vi "Teste-Circulos.vi"() -> ()   [LabVIEW 2014]
doc: "Newport Motion Controler\nThis VI test a Group\n\nAndré Romero - 2022\nandretec@ifsc.usp.br"
uses:
  <vilib>/Platform/TimedLoop/XDataNode/timing_clust.ctl
  <vilib>/Platform/TimedLoop/XDataNode/nitl_modes.ctl
  <vilib>/Platform/TimedLoop/XDataNode/wakeup.ctl
  <vilib>/Platform/TimedLoop/XDataNode/XDataNode.xnode
  <userlib>/Newport ESP301/Newport ESP301.lvlib
  <vilib>/Platform/TimedLoop/XDataNode/XDNodeRunTimeDep.lvlib
panel:
  out "Position (units) 4":dbl format="%.6g"
  out "Position (units) 3":dbl format="%.6g"
  out "Position (units) 2":dbl format="%.6g"
  out "Position (units)":dbl format="%.6g"
  in  "arc sweep angle":dbl=360.0 format="%#_13g"
  in  "Second coordonate of arc center":dbl format="%#_13g"
  in  "first coordonate of arc":dbl=0.1 format="%#_13g"
  in  "Stop Button":bool
  out "error out":errorcluster
  out "Y":dbl format="%.2g"
  out "X":dbl=-0.2115 format="%.2f"
  out "XY Graph":cluster{dbl[], dbl[]}(graph)={[-0.0005, -0.027, -0.0515, -0.076, -0.1, -0.1235, -0.146, -0.1675, -0.1885, -0.207, -0.2255, -0.242, -0.257, -0.2705, -0.2815, -0.2915, -0.2995, -0.3055, -0.3095, -0.3115, -0.312, -0.311, -0.3055, -0.2995, -0.292, -0.282, -0.2705, -0.257, -0.242, -0.2255, -0.2075, -0.1885, -0.168, -0.146, -0.1235, -0.1005, -0.076, -0.052, -0.0275, -0.0025, 0.023, 0.0475, 0.0725, 0.0965, 0.1195, 0.142, 0.164, 0.185, 0.204, 0.2225, 0.239, 0.2545, 0.268, 0.2795, 0.2895, 0.2975, 0.3045, 0.3085, 0.311, 0.3115, 0.311, 0.3065, 0.3, 0.2925, 0.283, 0.2715, 0.2585, 0.244, 0.2275, 0.2095, 0.191, 0.1705, 0.149, 0.126, 0.1035, 0.079, 0.0545, 0.03, 0.0055, -0.0015, -0.0005, 0.0, 0.0, 0.0, 0.0, 0.0, 0.0, 0.0, 0.0, 0.0, 0.0, 0.0, 0.0, 0.0, 0.0, 0.0, 0.0, 0.0, 0.0, 0.0, 0.0, 0.0, 0.0, 0.0, 0.0, 0.0, 0.0, 0.0, 0.0, 0.0, 0.0, 0.0, 0.0, 0.0, 0.0, 0.0, 0.0, 0.0, 0.0, 0.0, 0.0, 0.0, 0.0, 0.0, 0.0, 0.0, 0.0, 0.0, 0.0, 0.0, 0.0, 0.0, 0.0, 0.0, 0.0, 0.0, 0.0, 0.0, 0.0, 0.0, 0.0, 0.0, 0.0, 0.0, 0.0, 0.0, 0.0, 0.0, 0.0, 0.0, 0.0, 0.0, 0.0, 0.0, 0.0, 0.0, 0.0, 0.0, 0.0, 0.0, 0.0, 0.0, 0.0, 0.0, 0.0, 0.0, 0.0, 0.0, 0.0, 0.0, 0.0, 0.0, 0.0, 0.0, 0.0, 0.0, 0.0, 0.0, 0.0, 0.0, 0.0, 0.0, 0.0, 0.0, 0.0, 0.0, 0.0, 0.0, 0.0, 0.0, 0.0, 0.0, 0.0, 0.0, 0.0, 0.0, 0.0, 0.0, 0.0, 0.0, 0.0, 0.0, 0.0, 0.0, 0.0, 0.0, 0.0, 0.0, 0.0, 0.0, 0.0, 0.0, 0.0, 0.0, 0.0, 0.0, 0.0, 0.0, 0.0, 0.0, 0.0, 0.0, 0.0, 0.0, 0.0, 0.0, 0.0, 0.0, 0.0, 0.0, 0.0, 0.0, 0.0, 0.0, 0.0, 0.0, 0.0, 0.0, 0.0, 0.0, 0.0, 0.0, 0.0, 0.0, 0.0, 0.0, 0.0, 0.0, 0.0, 0.0, 0.0, 0.0, 0.0, 0.0, 0.0, 0.0, 0.0, 0.0, 0.0, 0.0, 0.0, 0.0, 0.0, 0.0, 0.0, 0.0, 0.0, 0.0, 0.0, 0.0, 0.0, 0.0, 0.0, 0.0, 0.0, 0.0, 0.0, 0.0, 0.0, 0.0, 0.0, 0.0, 0.0, 0.0, 0.0, 0.0, 0.0, 0.0, 0.0, 0.0, 0.0, 0.0, 0.0, 0.0, 0.0, 0.0, 0.0, 0.0, 0.0, 0.0, 0.0, 0.0, 0.0, 0.0, 0.0, 0.0, 0.0, 0.0, 0.0, 0.0, 0.0, 0.0, 0.0, 0.0, 0.0, 0.0, 0.0, 0.0, 0.0, 0.0, 0.0, 0.0, 0.0, 0.0, 0.0, 0.0, 0.0, 0.0, 0.0, 0.0, 0.0, 0.0, 0.0, 0.0, 0.0, 0.0, 0.0, 0.0, 0.0, 0.0, 0.0, 0.0, 0.0, 0.0, 0.0, 0.0, 0.0, 0.0, 0.0, 0.0, 0.0, 0.0, 0.0, 0.0, 0.0, 0.0, 0.0, 0.0, 0.0, 0.0, 0.0, 0.0, 0.0, 0.0, 0.0, 0.0, 0.0], [-0.2115, -0.211, -0.2075, -0.202, -0.195, -0.1855, -0.175, -0.1625, -0.148, -0.132, -0.115, -0.096, -0.0765, -0.055, -0.033, -0.01, 0.0135, 0.038, 0.0625, 0.0875, 0.1125, 0.1375, 0.1625, 0.1865, 0.21, 0.233, 0.2555, 0.2765, 0.2965, 0.3155, 0.3325, 0.349, 0.363, 0.3755, 0.386, 0.3955, 0.4025, 0.4075, 0.4105, 0.412, 0.412, 0.41, 0.4035, 0.3965, 0.3875, 0.3775, 0.365, 0.351, 0.3355, 0.318, 0.2995, 0.2795, 0.2585, 0.2365, 0.214, 0.19, 0.166, 0.1415, 0.1165, 0.0915, 0.0665, 0.042, 0.0175, -0.007, -0.0295, -0.0515, -0.073, -0.093, -0.112, -0.13, -0.146, -0.1605, -0.173, -0.184, -0.1935, -0.201, -0.2065, -0.2095, -0.2115, -0.2115, -0.2115, -0.2115, -0.2115, -0.2115, -0.2115, -0.2115, -0.212, -0.2115, -0.2115, -0.2115, -0.2115, -0.2115, -0.2115, -0.2115, -0.2115, -0.2115, -0.2115, -0.2115, -0.2115, -0.2115, -0.2115, -0.2115, -0.2115, -0.2115, -0.2115, -0.2115, -0.2115, -0.2115, -0.2115, -0.2115, -0.2115, -0.2115, -0.2115, -0.2115, -0.2115, -0.2115, -0.2115, -0.2115, -0.2115, -0.2115, -0.2115, -0.2115, -0.2115, -0.2115, -0.2115, -0.2115, -0.2115, -0.2115, -0.2115, -0.2115, -0.2115, -0.2115, -0.2115, -0.2115, -0.2115, -0.2115, -0.2115, -0.2115, -0.2115, -0.2115, -0.2115, -0.2115, -0.2115, -0.2115, -0.2115, -0.2115, -0.2115, -0.2115, -0.2115, -0.2115, -0.2115, -0.2115, -0.2115, -0.2115, -0.2115, -0.2115, -0.2115, -0.2115, -0.2115, -0.2115, -0.2115, -0.2115, -0.2115, -0.2115, -0.2115, -0.2115, -0.2115, -0.2115, -0.2115, -0.2115, -0.2115, -0.2115, -0.2115, -0.2115, -0.2115, -0.2115, -0.2115, -0.2115, -0.2115, -0.2115, -0.2115, -0.2115, -0.2115, -0.2115, -0.2115, -0.2115, -0.2115, -0.2115, -0.2115, -0.2115, -0.2115, -0.2115, -0.2115, -0.2115, -0.2115, -0.2115, -0.2115, -0.2115, -0.2115, -0.2115, -0.2115, -0.2115, -0.2115, -0.2115, -0.2115, -0.2115, -0.2115, -0.2115, -0.2115, -0.2115, -0.2115, -0.2115, -0.2115, -0.2115, -0.2115, -0.2115, -0.2115, -0.2115, -0.2115, -0.2115, -0.2115, -0.2115, -0.2115, -0.2115, -0.2115, -0.2115, -0.2115, -0.2115, -0.2115, -0.2115, -0.2115, -0.2115, -0.2115, -0.2115, -0.2115, -0.2115, -0.2115, -0.2115, -0.2115, -0.2115, -0.2115, -0.2115, -0.2115, -0.2115, -0.2115, -0.2115, -0.2115, -0.2115, -0.2115, -0.2115, -0.2115, -0.2115, -0.2115, -0.2115, -0.2115, -0.2115, -0.2115, -0.2115, -0.2115, -0.2115, -0.2115, -0.2115, -0.2115, -0.2115, -0.2115, -0.2115, -0.2115, -0.2115, -0.2115, -0.2115, -0.2115, -0.2115, -0.2115, -0.2115, -0.2115, -0.2115, -0.2115, -0.2115, -0.2115, -0.2115, -0.2115, -0.2115, -0.2115, -0.2115, -0.2115, -0.2115, -0.2115, -0.2115, -0.2115, -0.2115, -0.2115, -0.2115, -0.2115, -0.2115, -0.2115, -0.2115, -0.2115, -0.2115, -0.2115, -0.2115, -0.2115, -0.2115, -0.2115, -0.2115, -0.2115, -0.2115, -0.2115, -0.2115, -0.2115, -0.2115, -0.2115, -0.2115, -0.2115, -0.2115, -0.2115, -0.2115, -0.2115, -0.2115, -0.2115, -0.2115, -0.2115, -0.2115, -0.2115, -0.2115, -0.2115, -0.2115, -0.2115, -0.2115, -0.2115, -0.2115, -0.2115, -0.2115, -0.2115, -0.2115, -0.2115, -0.2115, -0.2115, -0.2115, -0.2115, -0.2115, -0.2115, -0.2115, -0.2115, -0.2115, -0.2115, -0.2115, -0.2115, -0.2115, -0.2115, -0.2115, -0.2115, -0.2115, -0.2115, -0.2115, -0.2115, -0.2115, -0.2115, -0.2115, -0.2115, -0.2115, -0.2115, -0.2115, -0.2115, -0.2115, -0.2115, -0.2115, -0.2115]}
  in  "Velocity":dbl=0.1
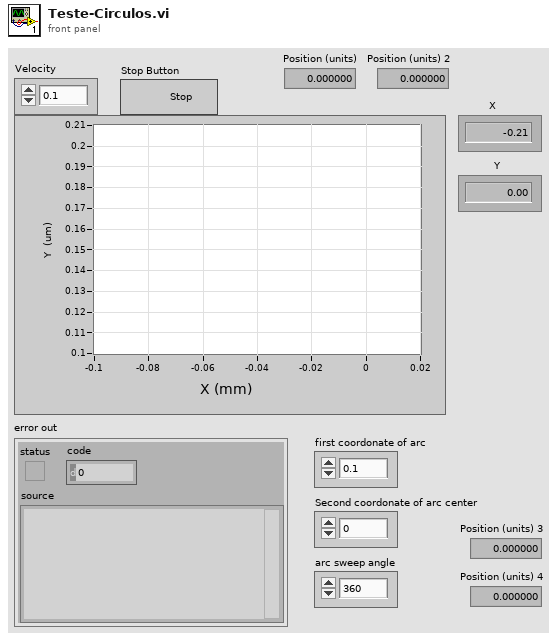
[diagram p1: front panel]
types:
  T1 = typedef "XDNodeRunTimeDep.lvlib/timing_clust.ctl" = cluster{"Expected End [f-1]":u64, "Actual End [f-1]":u64, "Finished Late? [f-1]":bool, "Expected End [i-1]":u64, "Actual End [i-1]":u64, "Finished Late? [i-1]":bool, "Expected Start [i]":u64, "Actual Start [i]":u64, "Expected Start [f]":u64, "Actual Start [f]":u64, "Source Name":string, "Structure Name":string, "Period":i64, "Deadline":i64, "Offset":i64, "Start":i64, "Priority":i32, "Timeout":i32, "Mode":T2, "Wakeup Reason":T3, "Error":errorcluster, "Source Type":string, "Secondary Source Type":string, "Global End Time":u64, "Global Start Time":u64, "Frame Duration":u64, "Iteration Duration":u64, "Assigned CPU":i32, "I/O Scan Engine Mode":u32}
  T2 = typedef "XDNodeRunTimeDep.lvlib/nitl_modes.ctl" = enum32{"No Change", "Process missed periods, maintain original phase", "Discard missed periods, maintain original phase", "Process missed periods, ignore original phase", "Discard missed periods, ignore original phase"}
  T3 = typedef "XDNodeRunTimeDep.lvlib/wakeup.ctl" = enum32{"Normal", "Aborted", "Asynchronous wakeup", "Timing source error", "Timed loop error", "Timeout"}
  T4 = cluster{"first coordonate of arc":dbl, "Second coordonate of arc center":dbl, "arc sweep angle":dbl}
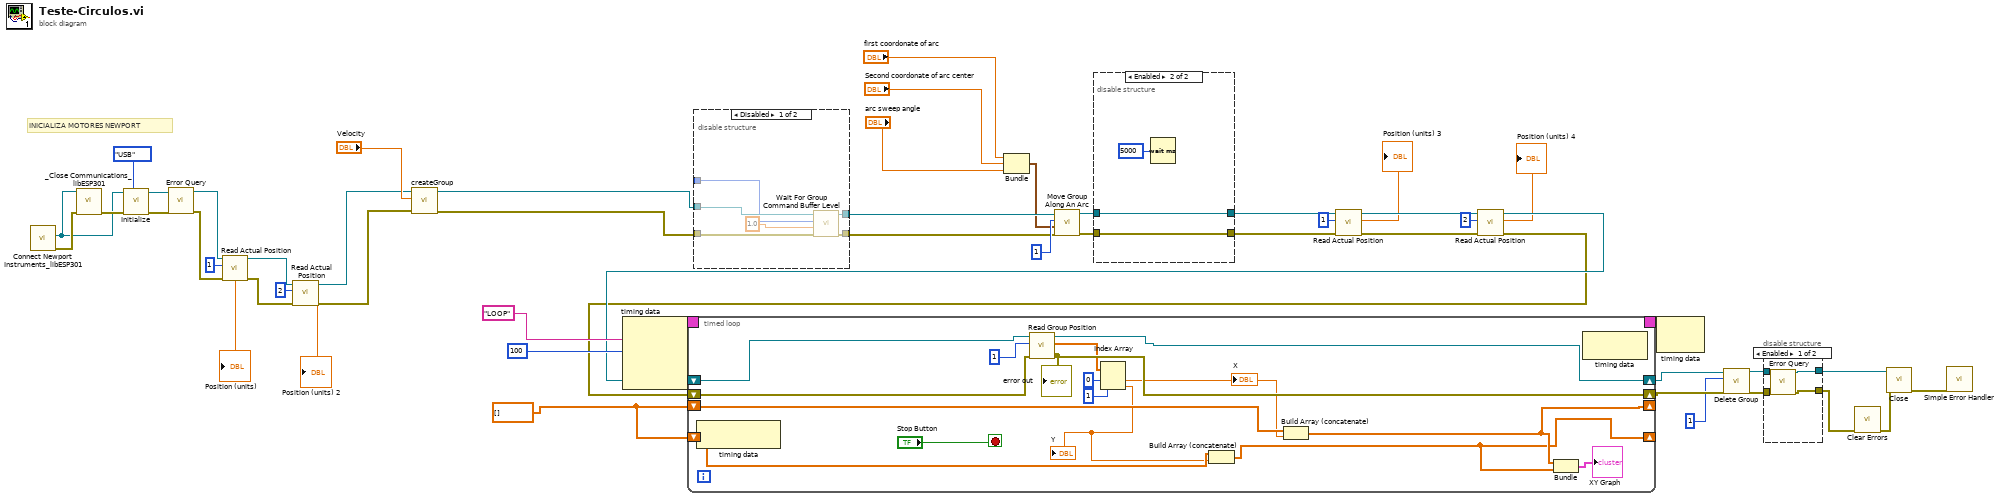
[diagram p0: block diagram]
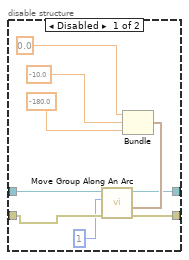
[diagram p2: hidden frame]
diagram:
  w31 = dbl[] []
  # "INICIALIZA MOTORES NEWPORT"
  n1 = call <userlib>:"Connect Newport Instruments_libESP301.vi"() -> ("error (duplicate)"=w50:errorcluster, "VISA resource name (duplicate)"=w49:refnum<visa-resource-name>)  [unwired: 7 in, 3 out]
  n2 = call <userlib>:"_Close Communications_libESP301.vi"("Instrument Channel"=w49, "error in (no error)"=w50) -> ("error out"=w52:errorcluster)  [unwired: 13 in]
  n3 = call <userlib>:"Initialize.vi"("VISA resource name"=w49, "error in (no error)"=w52, "Serial Link (RS232)"=enum16{"RS232", "USB"}."USB") -> ("VISA resource name out"=w48:refnum<visa-resource-name>, "error out"=w47:errorcluster)  [unwired: 6 in]
  n4 = call <userlib>:"Error Query.vi"("error in (no error)"=w47, "VISA resource name"=w48) -> ("error out"=w15:errorcluster, "VISA resource name out"=w20:refnum<visa-resource-name>)  [unwired: 2 in, 2 out]
  n5 = call <userlib>:"Read Actual Position.vi"("error in (no error)"=w15, "Axis (1)"=1, "VISA resource name"=w20) -> ("error out"=w18:errorcluster, "Position (units)"=→"Position (units)":dbl, "VISA resource name out"=w19:refnum<visa-resource-name>)  [unwired: 2 in]
  n6 = call <userlib>:"Read Actual Position.vi"("error in (no error)"=w18, "Axis (1)"=2, "VISA resource name"=w19) -> ("error out"=w16:errorcluster, "Position (units)"=→"Position (units) 2":dbl, "VISA resource name out"=w17:refnum<visa-resource-name>)  [unwired: 2 in]
  n7 = call "createGroup.vi"("error in (no error)"=w16, "Velocity"="Velocity", "VISA Refnum in"=w17) -> ("error out"=w44:errorcluster, "VISA Refnum out"=w45:refnum<visa-resource-name>)  [unwired: 7 in]
  n8 = node-c288("LOOP" ("Structure Name"), i64 100 ("Period")) -> (w35:T1)  [unwired: 2 in]
  n9 = disable-structure shown="Disabled" {
    disable-tunnel: w45 -> [w58 w60]
    disable-tunnel: w44 -> [w57 w59]
    disable-tunnel: [w56 w60] -> w43
    disable-tunnel: [w55 w59] -> w42
    disable-tunnel: _ -> [w53 _]
    frame Disabled {
      n10 = call <userlib>:"Wait For Group Command Buffer Level.vi"("error in (no error)"=w57, "level in group via point buffer"=1.0, "Group Number (1)"=w53, "VISA resource name"=w58) -> ("error out"=w55:errorcluster, "VISA resource name out"=w56:refnum<visa-resource-name>)  [unwired: 2 in]
    }
    frame Enabled {
    }
  }
  n11 = Bundle("first coordonate of arc"="first coordonate of arc", "Second coordonate of arc center"="Second coordonate of arc center", "arc sweep angle"="arc sweep angle") -> (w36:T4)  [unwired: 1 in]
  n12 = call <userlib>:"Move Group Along An Arc.vi"("error in (no error)"=w42, "Arc  Parameters"=w36, "Group Number (1)"=1, "VISA resource name"=w43) -> ("error out"=w40:errorcluster, "VISA resource name out"=w41:refnum<visa-resource-name>)  [unwired: 2 in]
  n13 = disable-structure shown="Enabled" {
    disable-tunnel: w41 -> [w69 w72]
    disable-tunnel: w40 -> [w68 w71]
    disable-tunnel: [w62 w72] -> w10
    disable-tunnel: [w61 w71] -> w9
    frame Disabled {
      n14 = Bundle(0.0, -10.0, -180.0) -> (w64:cluster{dbl, dbl, dbl})  [unwired: 1 in]
      n15 = call <userlib>:"Move Group Along An Arc.vi"("error in (no error)"=w68, "Arc  Parameters"=w64, "Group Number (1)"=1, "VISA resource name"=w69) -> ("error out"=w61:errorcluster, "VISA resource name out"=w62:refnum<visa-resource-name>)  [unwired: 2 in]
    }
    frame Enabled {
      n16 = Wait (ms)(milliseconds to wait=u32 5000) -> ()  [unwired: 1 out]
    }
  }
  n17 = call <userlib>:"Read Actual Position.vi"("error in (no error)"=w9, "Axis (1)"=1, "VISA resource name"=w10) -> ("error out"=w7:errorcluster, "Position (units)"=→"Position (units) 3":dbl, "VISA resource name out"=w8:refnum<visa-resource-name>)  [unwired: 2 in]
  n18 = call <userlib>:"Read Actual Position.vi"("error in (no error)"=w7, "Axis (1)"=2, "VISA resource name"=w8) -> ("error out"=w5:errorcluster, "Position (units)"=→"Position (units) 4":dbl, "VISA resource name out"=w6:refnum<visa-resource-name>)  [unwired: 2 in]
  n19 = timed-loop {
    timing: w35 -> [_]
    timing-out: [_] -> w34
    shift-right: [w83] -> w26
    shift-left: w6 -> [w85]
    shift-right: [w82] -> w25
    shift-left: w5 -> [w84]
    shift-right: [w74] -> _
    shift-left: w31 -> [w88]
    shift-right: [w73] -> _
    shift-left: w31 -> [w87]
    stop <- "Stop Button" stop-if-true
    n20 = node-c288() -> ()  [unwired: 1 in, 1 out]
    n21 = call <userlib>:"Read Group Position.vi"("error in (no error)"=w84, "Group Number (1)"=1, "VISA resource name"=w85) -> ("error out"=w82:errorcluster, "Position (units)"=w79:dbl[], "VISA resource name out"=w83:refnum<visa-resource-name>)  [unwired: 2 in]
    "error out" <- w82
    n22 = Index Array(array=w79, index #1=0 ("index"), index #2=1 ("index")) -> (element #1=w78:dbl, element #2=w77:dbl)
    "Y" <- w77
    "X" <- w78
    n23 = Build Array (concatenate)(w87, w77) -> (w73:dbl[])
    n24 = Build Array (concatenate)(w88, w78) -> (w74:dbl[])
    n25 = Bundle(w74, w73) -> (→"XY Graph":cluster{dbl[], dbl[]})  [unwired: 1 in]
    n26 = node-c288() -> ()  [unwired: 1 in, 1 out]
  }
  n27 = node-c288(w34) -> ()  [unwired: 1 out]
  n28 = call <userlib>:"Delete Group.vi"("error in (no error)"=w25, "Group Number (1)"=1, "VISA resource name"=w26) -> ("error out"=w29:errorcluster, "VISA resource name out"=w30:refnum<visa-resource-name>)  [unwired: 3 in]
  n29 = disable-structure shown="Enabled" {
    disable-tunnel: w30 -> [w94 w96]
    disable-tunnel: w29 -> [w93 w95]
    disable-tunnel: [w92 w96] -> w28
    disable-tunnel: [w91 w95] -> w23
    frame Enabled {
      n30 = call <userlib>:"Error Query.vi"("error in (no error)"=w93, "VISA resource name"=w94) -> ("error out"=w91:errorcluster, "VISA resource name out"=w92:refnum<visa-resource-name>)  [unwired: 2 in, 2 out]
    }
    frame Disabled {
    }
  }
  n31 = call <vilib>:"Clear Errors.vi"("error in (no error)"=w23) -> ("error out"=w22:errorcluster)  [unwired: 5 in, 1 out]
  n32 = call <userlib>:"Close.vi"("error in (no error)"=w22, "VISA resource name"=w28) -> ("error out"=w27:errorcluster)  [unwired: 9 in]
  n33 = call <vilib>:"Simple Error Handler.vi"("error in (no error)"=w27) -> ()  [unwired: 4 in, 5 out]
